vi "FTW-Actor-Log-Error.vi"(0 "FTW Actor Instance":refnum<class "FTW-Actor-Instance.lvclass">, 5 "Explanation":string, 11 "Error to Log":errorcluster) -> (4 "FTW Actor Instance out":refnum<class "FTW-Actor-Instance.lvclass">, 6 "Exception Occurred?":bool, 8 "Exception":T1)   [LabVIEW 2015, in "FTW-Actor-Instance.lvclass"]
uses:
  FTW-Actor-Instance.lvclass
  error/FTW-ERR-ExceptionType.ctl
panel:
  # "Inputs"
  # "Outputs"
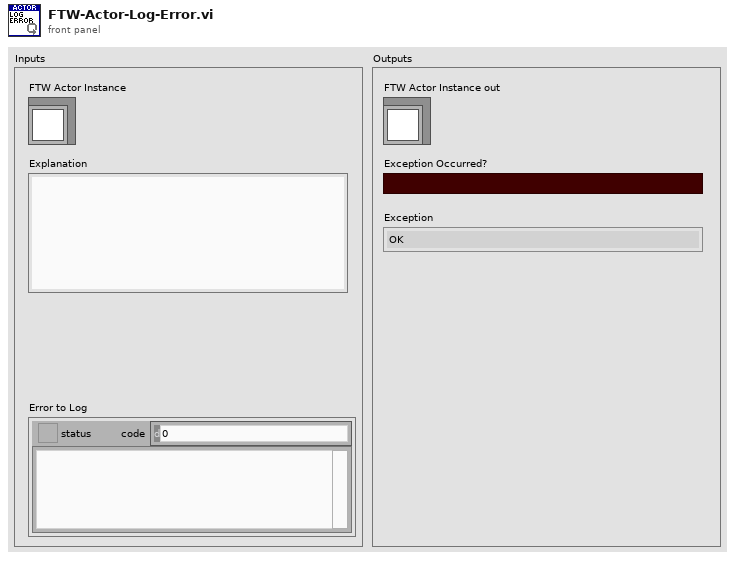
[diagram p1: front panel]
types:
  T1 = typedef "FTW-ERR-ExceptionType.ctl" = enum16{"OK", "Info", "Warning", "Error"}
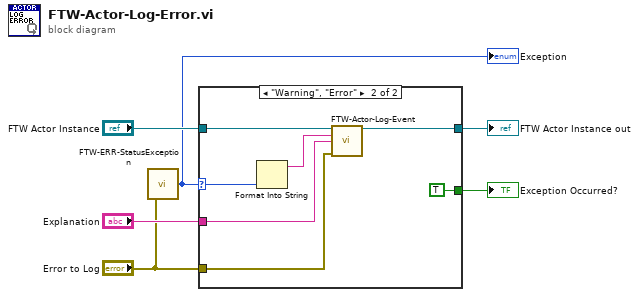
[diagram p0: block diagram]
diagram:
  n1 = call "FTW-ERR-StatusException.vi"("error to check"="Error to Log") -> ("Exception"=w1:T1)
  "Exception" <- w1
  n2 = case shown="\"Warning\", \"Error\"" w1 {
    selector: w1 -> [_ w10]
    tunnel: "Error to Log" -> [_ w8]
    tunnel: "FTW Actor Instance" -> [w7 w13]
    tunnel: [w7 w12] -> w5
    tunnel: [_ TRUE] -> w4
    tunnel: "Explanation" -> [_ w9]
    frame "OK", "Info" {
    }
    frame "Warning", "Error" {
      n3 = Format Into String(w10) -> (resulting string=w11:string)  [unwired: 3 in, 1 out]
      n4 = call-dynamic "FTW-Actor-Log-Event.vi"("FTW Actor Instance"=w13, "Event Type"=w11, "Event Data"=w9, "error in"=w8) -> ("FTW Actor Instance out"=w12:refnum<class "FTW-Actor-Instance.lvclass">)  [unwired: 10 in, 1 out]
    }
  }
  "FTW Actor Instance out" <- w5
  "Exception Occurred?" <- w4
